vi "Reset Output Protection.vi"(8 "error in (no error)":errorcluster, 10 "channel name (\"CHANNEL1\")":string="CHANNEL1", 11 "IVI_DCPwr in":refnum<class "IVI_DCPwr.lvclass">) -> (0 "error out":errorcluster, 3 "IVI_DCPwr out":refnum<class "IVI_DCPwr.lvclass">)   [LabVIEW 2013, in "IVI_DCPwr.lvlib" / "IVI_DCPwr.lvclass"]
doc: "This VI clears all output-protection conditions on the power supply."
uses:
  IVI_DCPwr.lvclass
  IVI_DCPwr.lvclass/IVI_DCPwr.ctl
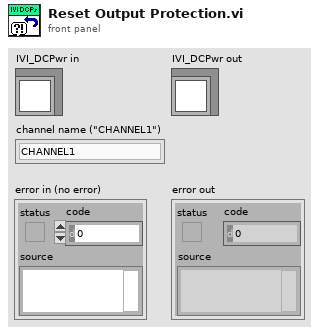
[diagram p1: front panel]
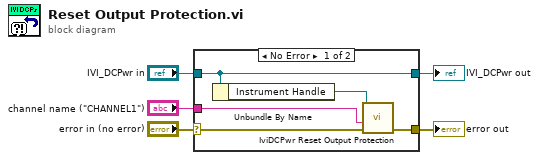
[diagram p0: block diagram]
diagram:
  n1 = case shown="No Error" "error in (no error)" {
    selector: "error in (no error)" -> [w8 w12]
    tunnel: [w7 w12] -> w4
    tunnel: [w10 w11] -> w2
    tunnel: "IVI_DCPwr in" -> [w10 w11]
    tunnel: "channel name (\"CHANNEL1\")" -> [w6 _]
    frame No Error {
      n2 = Unbundle By Name(w10) -> ("Instrument Handle"=w9:refnum<k15>)
      n3 = call <vilib>:"IviDCPwr Reset Output Protection.vi"("error in (no error)"=w8, "channel name (\"CHANNEL1\")"=w6, "instrument handle"=w9) -> ("error out"=w7:errorcluster)  [unwired: 7 in, 1 out]
    }
    frame Error {
    }
  }
  "error out" <- w4
  "IVI_DCPwr out" <- w2
